vi "Combine.vi"(11 "NewVal":u8[](array[numeric])) -> (3 "Data":u8[](array[numeric]))   [LabVIEW 2016]
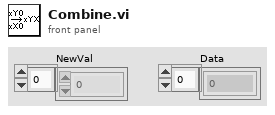
[diagram p1: front panel]
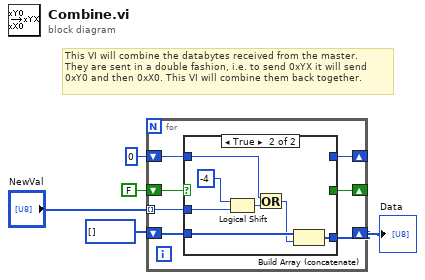
[diagram p0: block diagram]
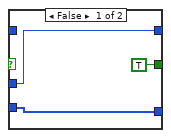
[diagram p2: hidden frame]
diagram:
  # "This VI will combine the databytes received from the master.\nThey are sent in a double fashion, i.e. to send 0xYX it will send \n0xY0 and then 0xX0. This VI will combine them back together."
  n1 = for {
    tunnel: "NewVal" -> [w12] mode=indexing
    shift-right: [w9] -> _
    shift-left: u8 0 -> [w10]
    shift-right: [w8] -> _
    shift-left: FALSE -> [w11]
    shift-right: [w6] -> w4
    shift-left: u8[] [] ("Data") -> [w7]
    n2 = case shown="True" w11 {
      tunnel: w12 -> [w15 w21]
      tunnel: w10 -> [_ w18]
      tunnel: [w15 _] -> w9
      tunnel: [TRUE _] -> w8
      tunnel: w7 -> [w13 w20]
      tunnel: [w13 w19] -> w6
      frame False {
      }
      frame True {
        n3 = Logical Shift(y=i8 -4 ("x"), x=w21) -> (x << y=w16:u8)
        n4 = Or(x=w18, y=w16) -> (x .or. y?=w17:u8)
        n5 = Build Array (concatenate)(w20, w17) -> (w19:u8[])
      }
    }
  }
  "Data" <- w4
